vi "Set Entry Sequence.vi"(8 "error in (no error)":errorcluster, 10 "Sequence":string, 11 "Execution in":refnum<class "Execution.lvclass">) -> (0 "error out":errorcluster, 3 "Execution out":refnum<class "Execution.lvclass">)   [LabVIEW 2020, in "HTS.lvlib" / "Execution.lvclass"]
uses:
  Execution.lvclass
  Execution.lvclass/Execution.ctl
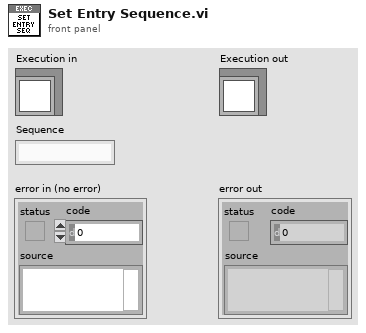
[diagram p1: front panel]
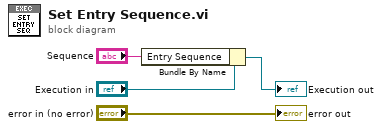
[diagram p0: block diagram]
diagram:
  n1 = Bundle By Name(cluster="Execution in", "Entry Sequence"="Sequence") -> (→"Execution out":refnum<class "Execution.lvclass">)
  "error out" <- "error in (no error)"
